vi "Create and Read AI.vi"(8 "error in":errorcluster, 10 "initial channel settings":T1[](array[typedef]), 11 "NI 9227 Test in":refnum<class "NI 9227 Test.lvclass">) -> (0 "error out":errorcluster, 2 "read channel settings":T1[](array[typedef]), 3 "NI 9227 Test out":refnum<class "NI 9227 Test.lvclass">)   [LabVIEW 2017, in "NI 9227 Test.lvclass"]
uses:
  NI 9227 Test.lvclass
  Scripting/Modules/Mode Classes/Controls/analog channel settings.ctl
  Scripting/Modules/NI 9227/NI 9227.lvclass
  Scripting/Scan Engine Scripting.lvlib
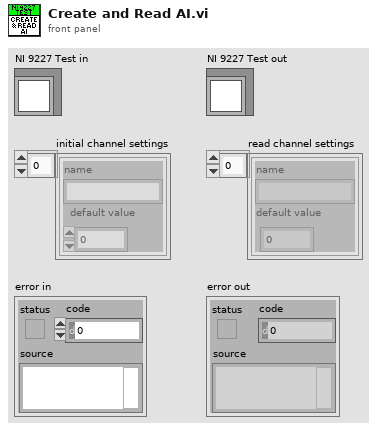
[diagram p1: front panel]
types:
  T1 = typedef "Scan Engine Scripting.lvlib/analog channel settings.ctl" = cluster{"name":string, "default value":dbl}
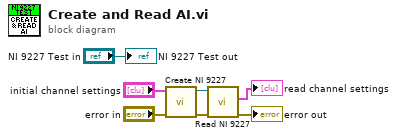
[diagram p0: block diagram]
diagram:
  n1 = call "Create NI 9227.vi"("error in"="error in", "channel settings"="initial channel settings") -> ("error out"=w2:errorcluster, "NI 9227 out"=w5:refnum<class "NI 9227.lvclass">)  [unwired: 8 in]
  n2 = call "Read NI 9227.vi"("error in"=w2, "NI 9227 in"=w5) -> ("error out"=→"error out":errorcluster, "channel settings"=→"read channel settings":T1[])  [unwired: 7 in, 1 out]
  "NI 9227 Test out" <- "NI 9227 Test in"
